vi "DataEntryProgramMarcoGonzalez.vi"() -> ()   [LabVIEW 2012]
doc: "VI will generate a one dimensional array with N elements filled with first names. The inputs should be the number of inputs (names) and each name. The output should be the name array and how many entries are in the array."
panel:
  in  "Name":string
  out "Array":string[](array[string])
  in  "# of Names Being Entered":dbl
  # "Marco Gonzalez\nEA3\n03 / 16 / 2017"
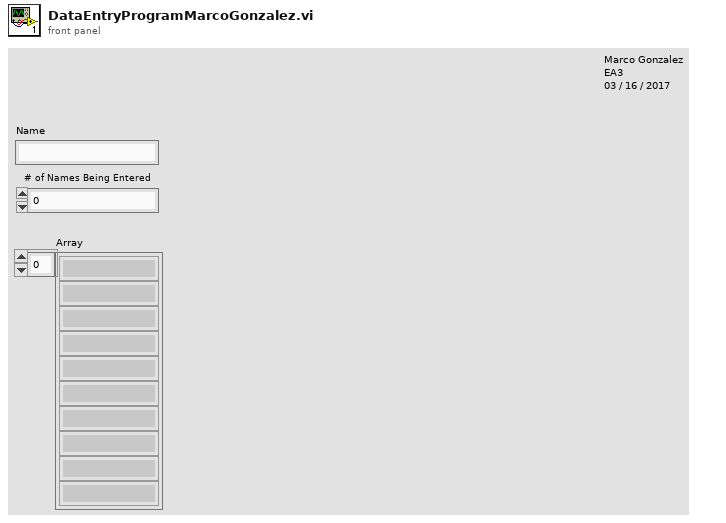
[diagram p1: front panel]
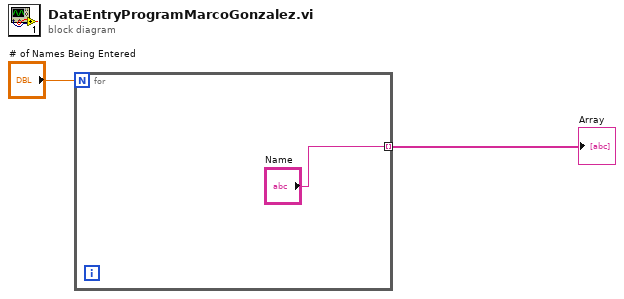
[diagram p0: block diagram]
diagram:
  n1 = for {
    N: "# of Names Being Entered" -> [_]
    tunnel: ["Name"] -> w1 mode=indexing
  }
  "Array" <- w1
